vi "Settings Dialog.vi"(0 "Settings in":T1, 3 "error in (no error)":errorcluster) -> (5 "FuzzyMap change?":bool, 7 "Settings out":T1, 8 "PID change?":bool, 9 "Cancelled?":bool, 10 "error out":errorcluster)   [LabVIEW 2016, in "Settings.lvlib"]
doc: "Dialog for selecting user specified settings."
uses:
  Settings.lvlib
  Settings.ctl
  Logging/Logging Configuration.ctl
  Acquisition/Hardware Configuration.ctl
  <vilib>/Utility/xml.llb/Write to XML File(string).vi
  Acquisition/Acquisition.lvlib
  Logging/Logging.lvlib
panel:
  in  "Cancel Button":bool
  in  "OK Button":bool
  in  "Tab Control":enum32{"Genaral", "Advance", "FuzzyMap"}(tab)
  in  "Haraware Config":cluster{"Bautrate":string, "VISA":T3}
  in  "Loging Config":T4
  in  "PID_parameter":T5
  in  "FuzzyMapTable":string[][](table)
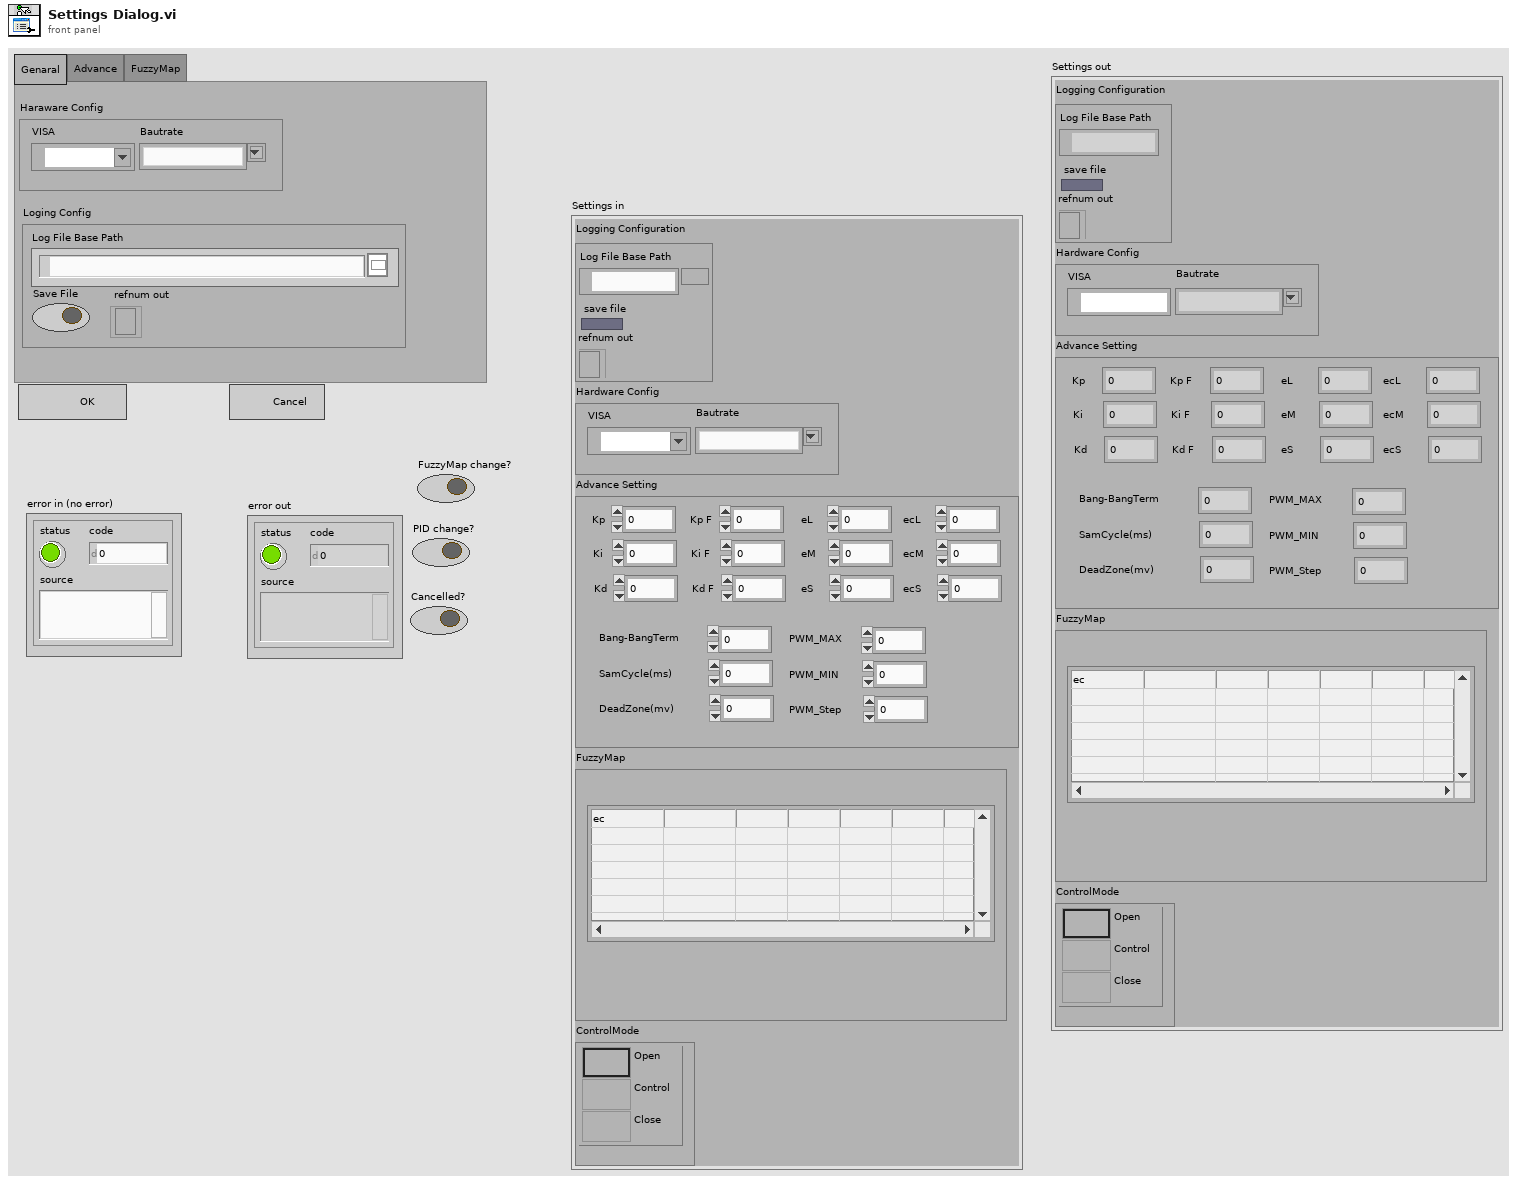
[diagram p1: front panel]
types:
  T1 = typedef "Settings.lvlib/Settings.ctl" = cluster{"Logging Configuration":T2, "Hardware Config":cluster{"Bautrate":string, "VISA":T3}, "Advance Setting":cluster{"PWM_Step":dbl, "PWM_MIN":dbl, "PWM_MAX":dbl, "DeadZone(mv)":dbl, "SamCycle(ms)":dbl, "Bang-BangTerm":dbl, "ecS":dbl, "ecM":dbl, "ecL":dbl, "eS":dbl, "eM":dbl, "eL":dbl, "Kd F":dbl, "Ki F":dbl, "Kp F":dbl, "Kd":dbl, "Ki":dbl, "Kp":dbl}, "FuzzyMap":cluster{"Table":string[][]}, "ControlMode":cluster{"Control":enum32{"1", "2", "4"}}}
  T2 = typedef "Logging.lvlib/Logging Configuration.ctl" = cluster{"Log File Base Path":path, "save file":bool, "refnum out":refnum<file>}
  T3 = typedef "Acquisition.lvlib/Hardware Configuration.ctl" = refnum<visa-resource-name>
  T4 = cluster{"Log File Base Path":path, "Save File":bool, "refnum out":refnum<file>}
  T5 = cluster{"PWM_Step":dbl, "PWM_MIN":dbl, "PWM_MAX":dbl, "DeadZone(mv)":dbl, "SamCycle(ms)":dbl, "Bang-BangTerm":dbl, "ecS":dbl, "ecM":dbl, "ecL":dbl, "eS":dbl, "eM":dbl, "eL":dbl, "Kd F":dbl, "Ki F":dbl, "Kp F":dbl, "Kd":dbl, "Ki":dbl, "Kp":dbl}
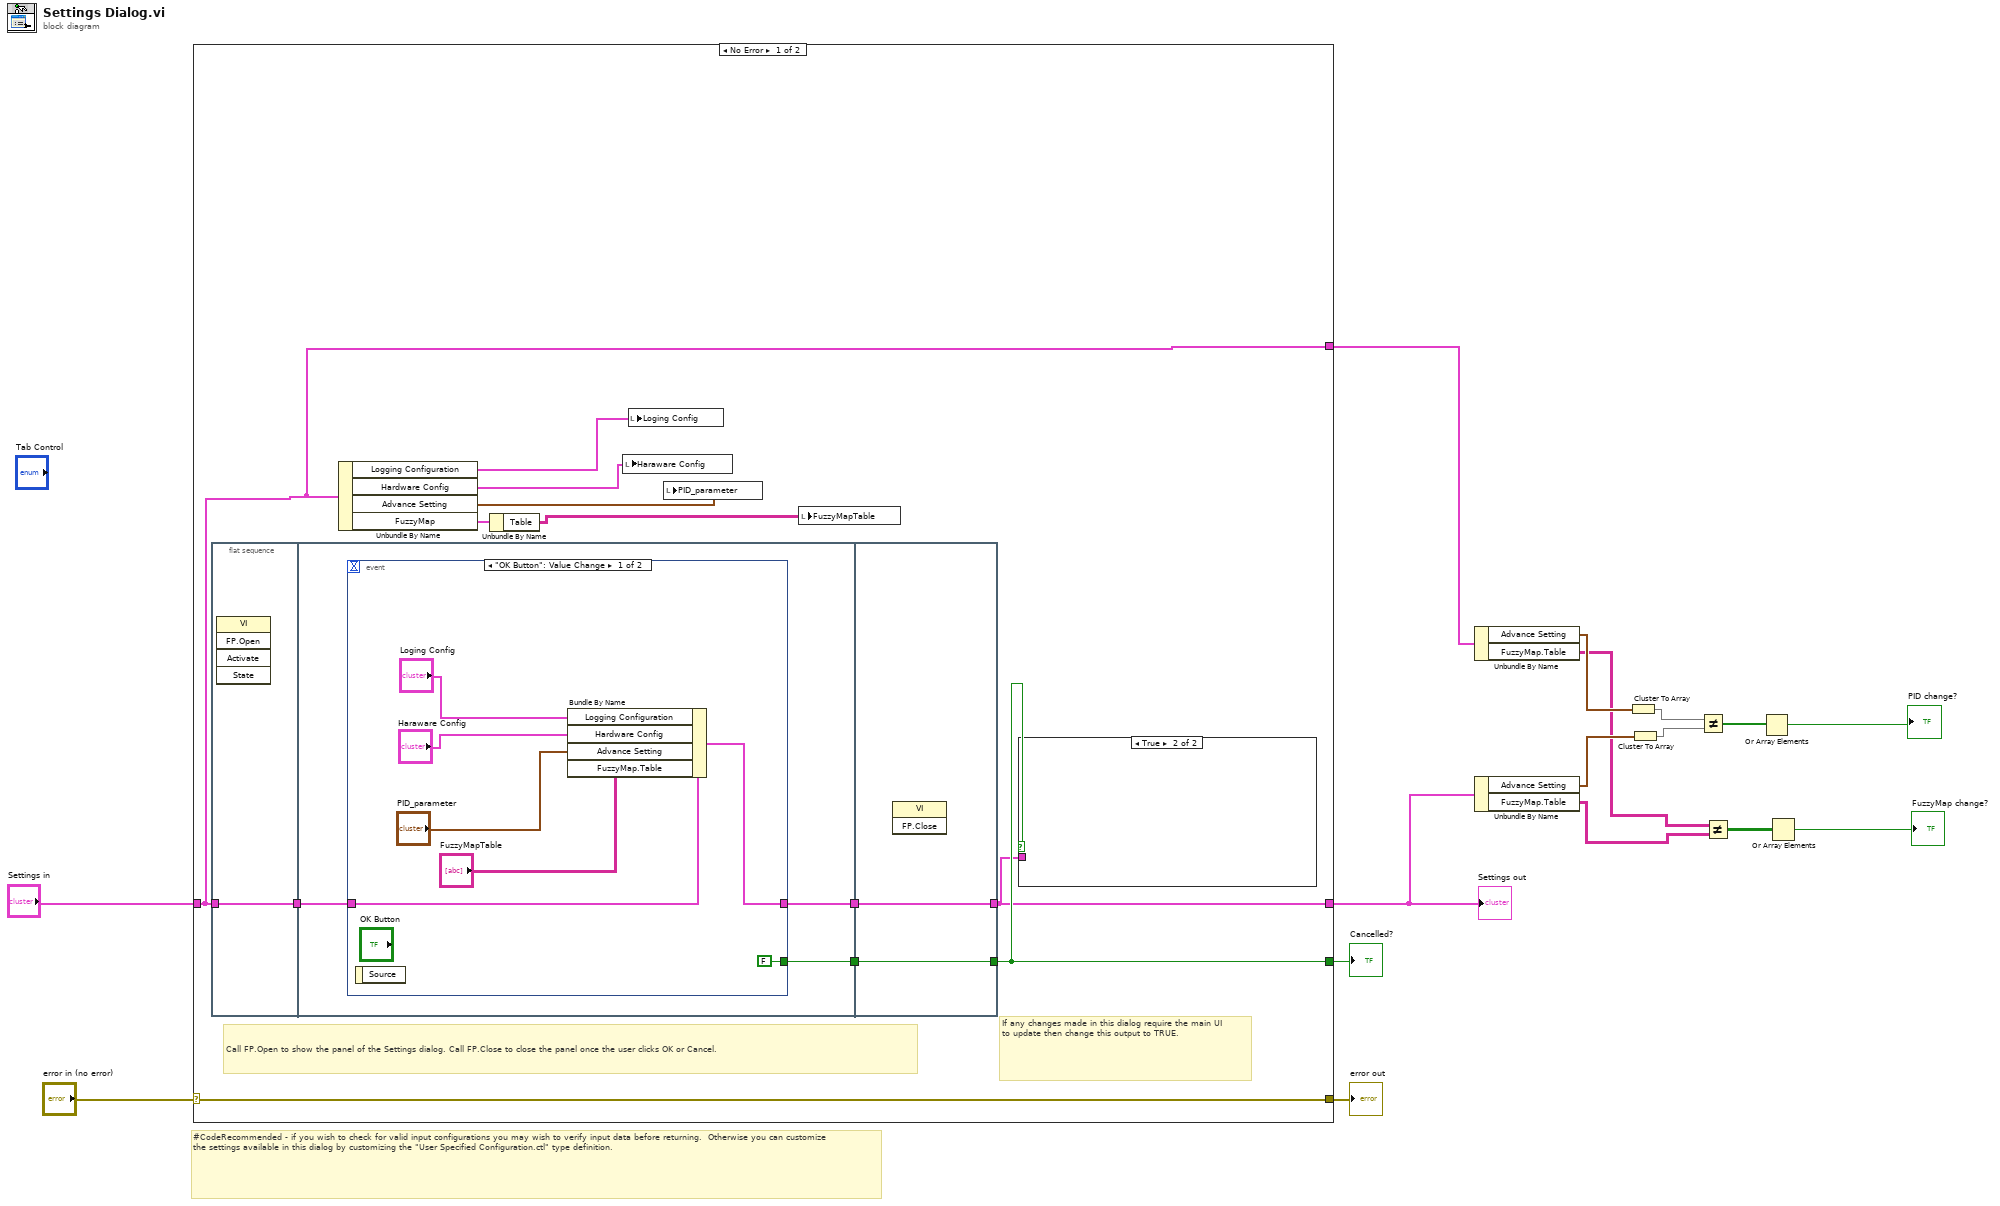
[diagram p0: block diagram]
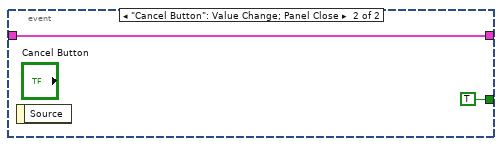
[diagram p2: hidden frame]
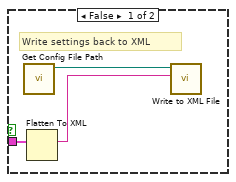
[diagram p3: hidden frame]
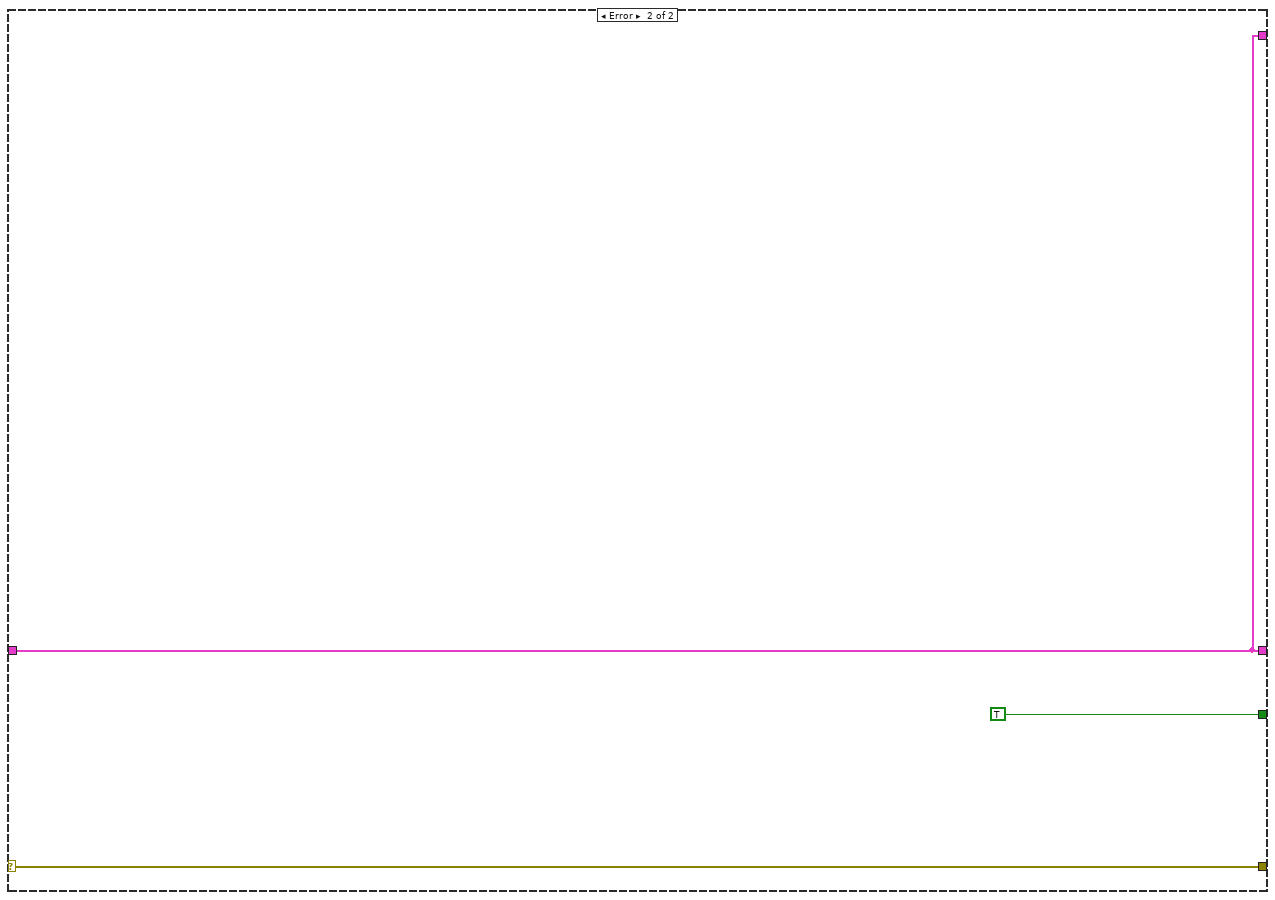
[diagram p4: hidden frame]
diagram:
  # "#CodeRecommended - if you wish to check for valid input configurations you may wish to verify input data before returning.  Otherwise you can customize the settings available in this dialog by customizing the \"User Specified Configuration.ctl\" type definition."
  n1 = case shown="No Error" "error in (no error)" {
    selector: "error in (no error)" -> [w28 w49]
    tunnel: [w28 w49] -> w15
    tunnel: "Settings in" -> [w17 w47]
    tunnel: [w26 w47] -> w11
    tunnel: [w27 TRUE ("UI Refresh Needed?")] -> w14
    tunnel: [w17 w47] -> w12
    frame No Error {
      # "Call FP.Open to show the panel of the Settings dialog. Call FP.Close to close the panel once the user clicks OK or Cancel."
      # "If any changes made in this dialog require the main UI to update then change this output to TRUE."
      n2 = flat-sequence {
        tunnel: w17 -> [w29]
        tunnel: [w29] -> w25
        tunnel: w25 -> [w30]
        tunnel: [w32] -> w24
        tunnel: [w31] -> w23
        tunnel: [w42] -> w26
        tunnel: [w43] -> w27
        tunnel: w24 -> [w43]
        tunnel: w23 -> [w42]
        frame #0 {
          n3 = invoke class="VI" method="FP.Open"() -> ()  [unwired: 5 in, 5 out]
        }
        frame #1 {
          n4 = event shown="[0] \"OK Button\": Value Change" {
            selector: _ -> [_ _]
            dyn-events: _ -> [_ _]
            timeout: _ -> [_ _]
            tunnel: [w37 w41] -> w31
            tunnel: w30 -> [w38 w41]
            tunnel: [FALSE ("UI Refresh Needed?") TRUE ("UI Refresh Needed?")] -> w32
            event "OK Button": Value Change {
              n5 = event-data() -> ()  [unwired: 1 in, 1 out]
              n6 = Bundle By Name(cluster=w38, "Logging Configuration"="Loging Config", "Hardware Config"="Haraware Config", "Advance Setting"="PID_parameter", "FuzzyMap.Table"="FuzzyMapTable") -> (w37:T1)
            }
            event "Cancel Button": Value Change; Panel Close {
              n7 = event-data() -> ()  [unwired: 1 in, 1 out]
            }
          }
        }
        frame #2 {
          n8 = invoke class="VI" method="FP.Close"() -> ()  [unwired: 3 in, 3 out]
        }
      }
      n9 = Unbundle By Name(w17) -> ("Logging Configuration"=w22:T2, "Hardware Config"=w21:cluster{"Bautrate":string, "VISA":T3}, "Advance Setting"=w20:T5, "FuzzyMap"=w19:cluster{"Table":string[][]})
      n10 = Unbundle By Name(w19) -> ("Table"=w18:string[][])
      n11 = local write "Haraware Config"(w21) -> ()
      n12 = local write "Loging Config"(w22) -> ()
      n13 = local write "PID_parameter"(w20) -> ()
      n14 = local write "FuzzyMapTable"(w18) -> ()
      n15 = case shown="True" w27 {
        tunnel: w26 -> [w45 _]
        frame False {
          # "Write settings back to XML"
          n16 = call "Get Config File Path.vi"() -> ("XML File Path"=w46:path)  [unwired: 10 in, 1 out]
          n17 = Flatten To XML(anything=w45) -> (xml string=w44:string)
          n18 = call-poly <vilib>:"Write to XML File.vi"("XML Input"=w44, "XML File Path"=w46) -> ()  [unwired: 7 in, 3 out]
        }
        frame True {
        }
      }
    }
    frame Error {
    }
  }
  "error out" <- w15
  "Cancelled?" <- w14
  "Settings out" <- w11
  n19 = Unbundle By Name(w12) -> ("Advance Setting"=w10:T5, "FuzzyMap.Table"=w4:string[][])
  n20 = Unbundle By Name(w11) -> ("Advance Setting"=w9:T5, "FuzzyMap.Table"=w3:string[][])
  n21 = Cluster To Array(cluster=w10) -> (array=w8:dbl[])
  n22 = Cluster To Array(cluster=w9) -> (array=w7:dbl[])
  n23 = Not Equal?(x=w8, y=w7) -> (x != y?=w6:bool[])
  n24 = Not Equal?(x=w4, y=w3) -> (x != y?=w2:bool[][])
  n25 = Or Array Elements(Boolean array=w6) -> (logical OR=→"PID change?":bool)
  n26 = Or Array Elements(Boolean array=w2) -> (logical OR=→"FuzzyMap change?":bool)
